vi "FFT_Processing.vi"(11 "scaled signals [EU]":waveform(dbl)[](array[waveform])) -> (0 "error out":errorcluster, 2 "peaks":cluster{"freq. or order":dbl, "value":dbl}[][](array[cluster]) {"value" format="%.2f"; "freq. or order" format="%.2f"}, 3 "magnitudes [dB EU]":cluster{"f0":dbl, "df":dbl, "magnitude":dbl[]}[](array[cluster]) {"magnitude" format="%.2p"; "df" format="%.2p"; "f0" format="%.2p"})   [LabVIEW 2023]
uses:
  <vilib>/addons/_NISVFA/_Subset FFT/SVFA FFT Spectrum Subset (Mag-Phase) (N Ch).vi
  <vilib>/addons/_NISVFA/_Spectrum Processing/SVFA Spectrum Peak Search (N Ch).vi
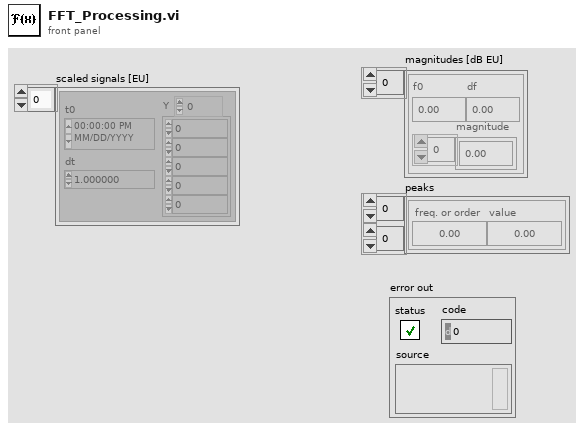
[diagram p1: front panel]
types:
  T1 = cluster{"single/multiple":enum16{"Multiple Peaks", "Single Max Peak"}, "threshold":dbl}
  T2 = cluster{"dB On (T)":bool, "unwrap phase (F)":bool, "convert to degree (T)":bool}
  T3 = cluster{"start frequency":dbl, "stop frequency":dbl}
  T4 = typedef "svc_Spectrum Info.ctl" = cluster{"channel name":string, "description":string, "x-axis units":T5, "spectral info":cluster{"spectrum type":T6, "linear/dB":enum16{"linear", "dB"}, "window":u16, "window size":i32, "FFT size":i32}, "engineering units":T7, "custom label":string, "dB reference [EU]":dbl, "peak units":enum16{"rms", "peak", "peak-peak"}, "weighting filter":T8, "spectral density?":bool, "unit label":string, "spectrum skewed?":bool, "complimentary spectrum units":T9}
  T5 = typedef "svc_X-Axis Units.ctl" = u16
  T6 = typedef "svc_Spectrum Type.ctl" = enum16{"FFT Spectrum [complex]", "Amplitude [Magnitude]", "Power [Magnitude^2]", "Cross Spectrum [complex]", "Frequency Response [Complex]"}
  T7 = typedef "svc_Engineering Units Text Ring.ctl" = u16
  T8 = typedef "svc_Weighting Filter Text Ring.ctl" = u16
  T9 = typedef "svc_Complimentary Spectrum Units.ctl" = enum16{"none", "radians", "degrees", "cycles", "imaginary"}
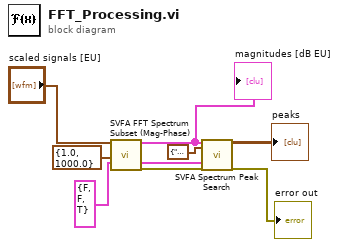
[diagram p0: block diagram]
diagram:
  n1 = call-poly <vilib>:"SVFA FFT Spectrum Subset (Mag-Phase).vi"("scaled signals [EU]"="scaled signals [EU]", "frequency range"=T3 {"start frequency"=1.0, "stop frequency"=1000.0}, "view"=T2 {"dB On (T)"=FALSE, "unwrap phase (F)"=FALSE, "convert to degree (T)"=TRUE}) -> ("magnitudes [dB EU]"=w9:cluster{"f0":dbl, "df":dbl, "magnitude":dbl[]}[], "spectrum info"=w8:T4[], "error out"=w7:errorcluster)  [unwired: 9 in, 5 out]
  "magnitudes [dB EU]" <- w9
  n2 = call-poly <vilib>:"SVFA Spectrum Peak Search.vi"("spectra"=w9, "peak search settings"=T1 {"single/multiple"=enum."Multiple Peaks", "threshold"=0.01}, "spectrum info"=w8, "error in (no error)"=w7) -> ("peaks"=→"peaks":cluster{"freq. or order":dbl, "value":dbl}[][], "error out"=→"error out":errorcluster)  [unwired: 11 in, 3 out]
